vi "Mouse Click Event.vi"() -> ()   [LabVIEW 2016]
panel:
  out "Plot.Plot Name":string
  out "Value":dbl
  out "Label.Text":string
  out "Waveform Chart 2":dbl(graph)
  out "Waveform Chart 1":dbl(graph)
  in  "stop":bool
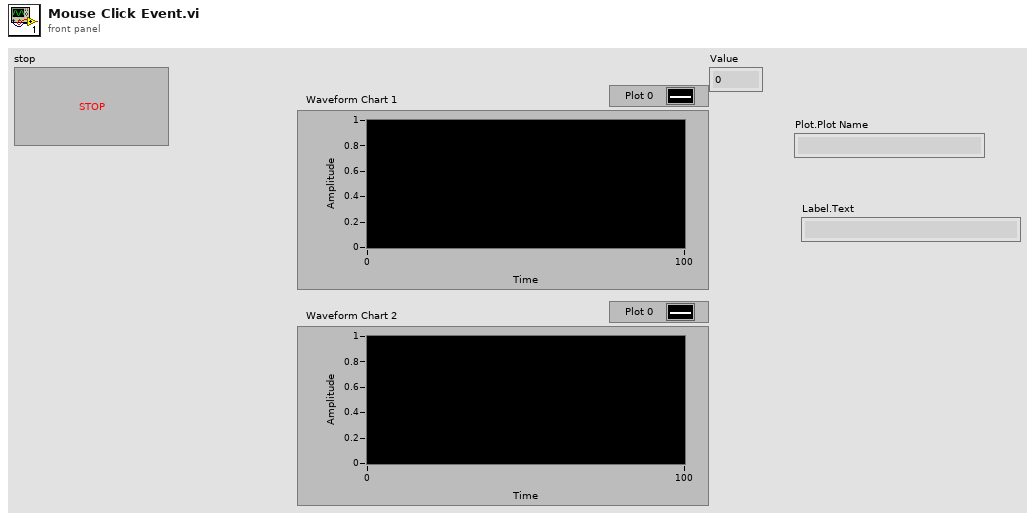
[diagram p1: front panel]
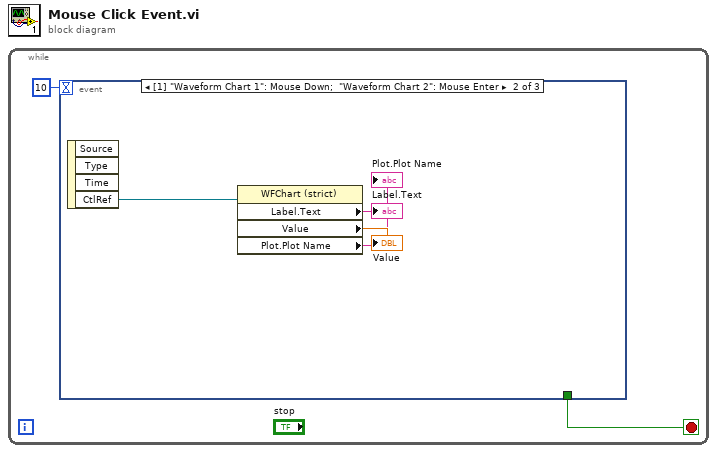
[diagram p0: block diagram]
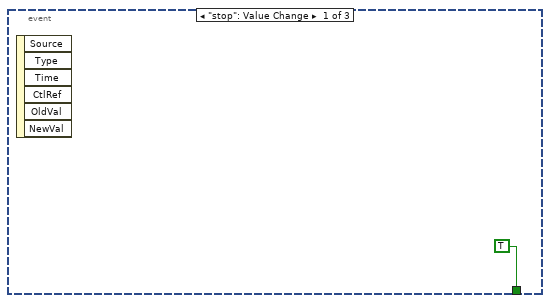
[diagram p2: hidden frame]
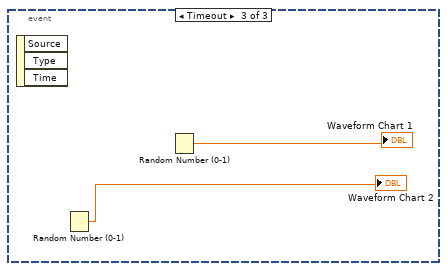
[diagram p3: hidden frame]
diagram:
  n1 = while {
    stop <- w2 stop-if-true
    n2 = event shown="[1] \"Waveform Chart 1\": Mouse Down;  \"Waveform Chart 2\": Mouse Enter" {
      selector: _ -> [_ _ _]
      dyn-events: _ -> [_ _ _]
      timeout: 10 -> [_ _ _]
      tunnel: [TRUE _ _] -> w2
      event "stop": Value Change {
        n3 = event-data() -> ()  [unwired: 1 in, 6 out]
      }
      event "Waveform Chart 1": Mouse Down; "Waveform Chart 2": Mouse Enter {
        n4 = event-data() -> ("CtlRef"=w7:refnum<vi>)  [unwired: 1 in, 3 out]
        n5 = property class="WFChart (strict)"(reference=w7) -> ("Label.Text"=→"Label.Text":string, "Value"=→"Value":dbl, "Plot.Plot Name"=→"Plot.Plot Name":string)  [unwired: 1 in, 2 out]
      }
      event Timeout {
        n6 = event-data() -> ()  [unwired: 1 in, 3 out]
        n7 = Random Number (0-1)() -> (number: 0 to 1=→"Waveform Chart 2":dbl)
        n8 = Random Number (0-1)() -> (number: 0 to 1=→"Waveform Chart 1":dbl)
      }
    }
  }
